vi "UI-Pore Diameter Detection.vi"(8 "error in (no error)":errorcluster caption="错误输入（无错误）", 11 "名称或相对路径":string="Template Program") -> (0 "error in (no error) 2":errorcluster caption="错误输入（无错误）")   [LabVIEW 2017]
uses:
  Picture/SaveButtom.ctl
  <vilib>/vision/Measure.llb/Edge Options.ctl
  <vilib>/vision/Measure.llb/Edge Polarity.ctl
  Global System.vi
  <vilib>/Utility/xml.llb/Read From XML File(string).vi
  <vilib>/Utility/xml.llb/Write to XML File(string).vi
panel:
  out "添加的路径 2":path
  out "计数器":dbl
  in  "启动200自动":bool
  out "孔径规格":T1
  out "原始图像 2":T2(plugin-control)
  in  "获取ROI":bool
  in  "GRR测试":bool
  in  "200测试":bool
  in  "采图按钮":bool
  in  "图像实时显示":bool
  out "添加的路径":path
  in  "刷新":bool
  in  "测试按钮":bool
  in  "保存按钮":bool
  in  "Main":enum32{"主参数", "计算圆心参数 ", "测试效果"}(tab)
  in  "ParamsUI":T3={"IsNorImage"=TRUE, "Exposure Values"=100289, "ImagePath"=path "C:/Users/hedongpo/Desktop/514-hdp/Alignment Assemble System/Test Picture/B/3.bmp"} caption="参数界面" {"Exposure Values" scale=0.0..200000.0}
  in  "ParamsUI 内圆":T7={"圆参数1"={"Search  Direction"=0, "Edge Options"={"Edge Polarity"=0, "Kernel Size"=3, "Width"=3, "Minimum Edge Strength"=50.0, "Interpolation Type"=enum."Bilinear Fixed", "Data Processing Method"=enum."Average"}, "Show Search Area"=TRUE, "Show Search Lines"=TRUE, "Show Edges Found"=TRUE, "Show Result"=TRUE, "Search Area Color"=65280, "Search Lines Color"=255, "Edge Locations Color"=16776960, "Result Color"=16711680, "Overlay Group Name"=""}, "圆参数"={"Process"=enum."Get First Edge", "Step Size"=1, "Max Pixel Radius"=3}, "圆环ROI设定"={"Center X"=1717, "Center Y"=1486, "Inner Radius"=327, "Outer Radius"=1645, "Start Angle"=0.0, "End Angle"=0.0}, "Show Search Area"=TRUE, "Show Search Lines"=TRUE, "Show Edges Found"=TRUE, "Show Result"=TRUE, "200次模板表格"=path "C:/Users/Administrator/Desktop/GRR模板/Test.xlsx", "GRR模板表格"=path "C:/Users/Administrator/Desktop/GRR模板/Test.xlsx", "孔径规格"={"孔径上限"="0.014", "孔径标准值"="1.1", "孔径下限"="0"}} caption="参数界面" {"圆环ROI设定"."End Angle" min=-90.0 max=90.0 step=1.0 format="%.2f"; "圆环ROI设定"."Start Angle" min=-90.0 max=90.0 step=1.0 format="%.2f"; "圆环ROI设定"."Center X" scale=0.0..1024.0; "圆参数1"."Search  Direction" items=["Outside to Inside", "Inside to Outside"]; "圆参数1"."Edge Options"."Edge Polarity" items=["All Edges", "Rising Edges", "Falling Edges"]; "圆参数1"."Edge Options"."Minimum Edge Strength" format="%.2f"; "圆参数1"."Edge Options"."Width" step=2; "圆参数1"."Edge Options"."Kernel Size" step=2}
  in  "测试历史记录":string[][](table)=[["", ""]]
  in  "测试结果":string[][](table)=[["", ""]]
  out "原始图像":T2(plugin-control)
  out "路径输出":path
  in  "Vision Paramter Save Buttom":T8
  out "system time":string
  in  "取消按钮":bool
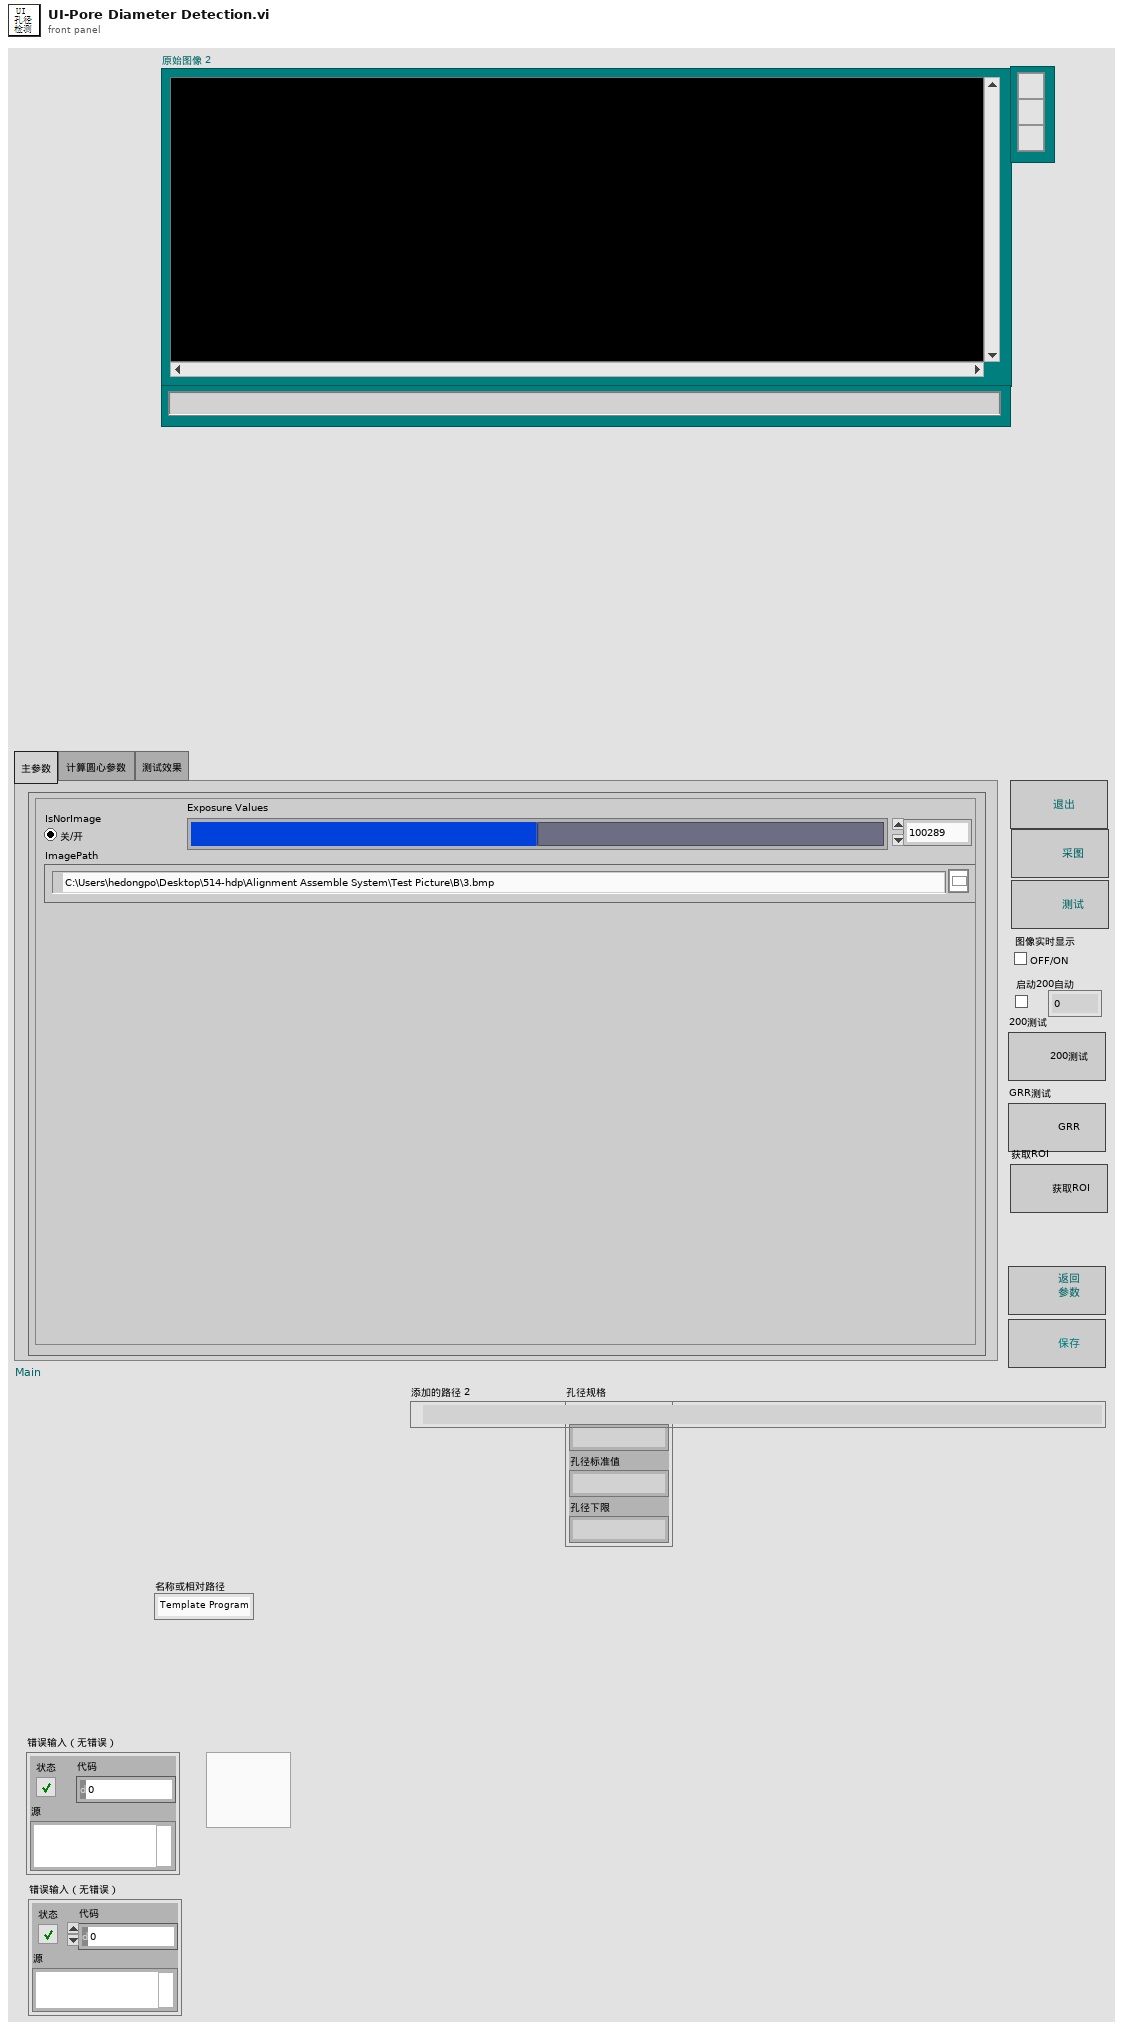
[diagram p1: front panel]
types:
  T1 = cluster{"孔径上限":string, "孔径标准值":string, "孔径下限":string}
  T2 = typedef "IMAQ Image.ctl" = refnum<image>
  T3 = cluster{"IsNorImage":bool, "Exposure Values":u32, "ImagePath":path}
  T4 = typedef "Edge Options.ctl" = cluster{"Edge Polarity":T5, "Kernel Size":u32, "Width":u32, "Minimum Edge Strength":sgl, "Interpolation Type":enum32{"Zero Order", "Bilinear", "Quadratic", "Cubic", "Bilinear Fixed"}, "Data Processing Method":enum32{"Average", "Median"}}
  T5 = typedef "Edge Polarity.ctl" = u32
  T6 = typedef "IMAQ Circle" = cluster{"Center X":i32, "Center Y":i32, "Inner Radius":i32, "Outer Radius":i32, "Start Angle":dbl, "End Angle":dbl}
  T7 = cluster{"圆参数1":cluster{"Search  Direction":u32, "Edge Options":T4, "Show Search Area":bool, "Show Search Lines":bool, "Show Edges Found":bool, "Show Result":bool, "Search Area Color":u32, "Search Lines Color":u32, "Edge Locations Color":u32, "Result Color":u32, "Overlay Group Name":string}, "圆参数":cluster{"Process":enum16{"Get First Edge", "Get First + Last Edge", "Get All Edges", "Get Best Edge"}, "Step Size":i32, "Max Pixel Radius":i32}, "圆环ROI设定":T6, "Show Search Area":bool, "Show Search Lines":bool, "Show Edges Found":bool, "Show Result":bool, "200次模板表格":path, "GRR模板表格":path, "孔径规格":cluster{"孔径上限":string, "孔径标准值":string, "孔径下限":string}}
  T8 = typedef "SaveButtom.ctl" = bool
  T9 = cluster{"index":i32, "this vi":refnum<vi>, "error out":errorcluster}
  T10 = cluster{"master data":string, "priority":u16, "secondary data":string[]}
  T11 = cluster{"case name":string[], "queue array":refnum<queue>[]}
  T12 = cluster{"Search  Direction":u32, "Edge Options":T4, "Show Search Area":bool, "Show Search Lines":bool, "Show Edges Found":bool, "Show Result":bool, "Search Area Color":u32, "Search Lines Color":u32, "Edge Locations Color":u32, "Result Color":u32, "Overlay Group Name":string}
  T13 = cluster{"Process":enum16{"Get First Edge", "Get First + Last Edge", "Get All Edges", "Get Best Edge"}, "Step Size":i32, "Max Pixel Radius":i32}
  T14 = typedef "ROI Descriptor" = cluster{"Global Rectangle":i32[], "Contours":cluster{"ID":enum32{"External", "Internal"}, "Type":u32, "Coordinates":i32[]}[]}
  T15 = cluster{"Center (Pixels)":cluster{"X":sgl, "Y":sgl}, "Radius (Pixels)":dbl, "Center (Real-World)":cluster{"X":sgl, "Y":sgl}, "Radius (Real-World)":dbl, "Roundness (Real-World)":dbl, "Average Strength":dbl, "Average SNR (dB)":dbl}
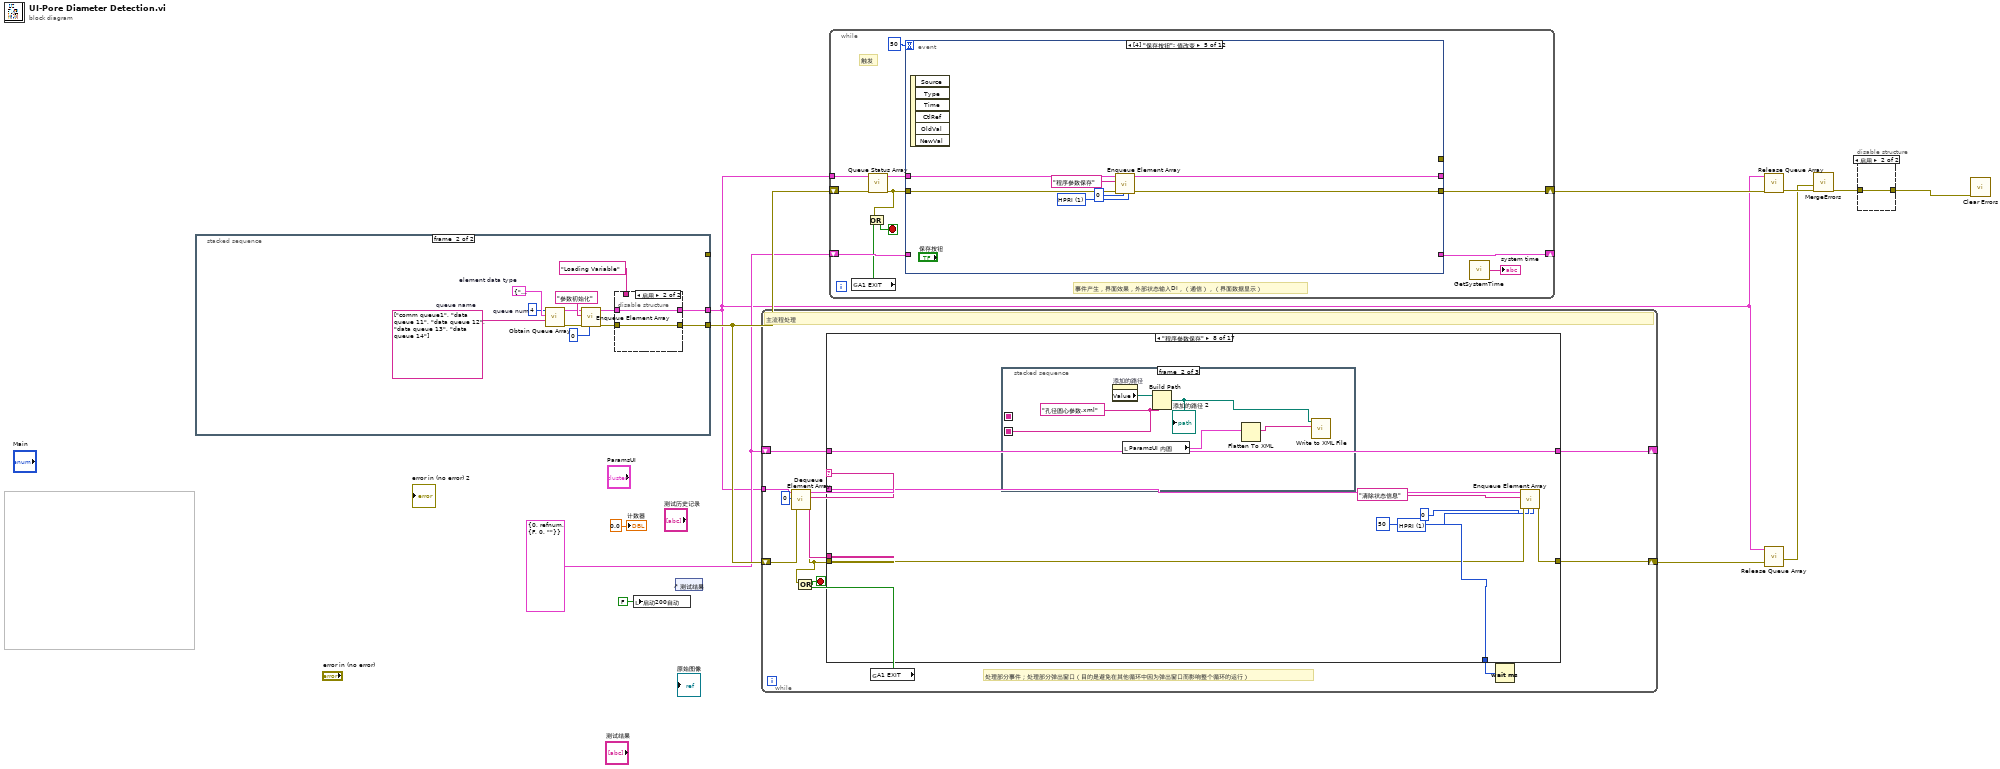
[diagram p0: block diagram]
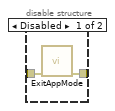
[diagram p2: hidden frame]
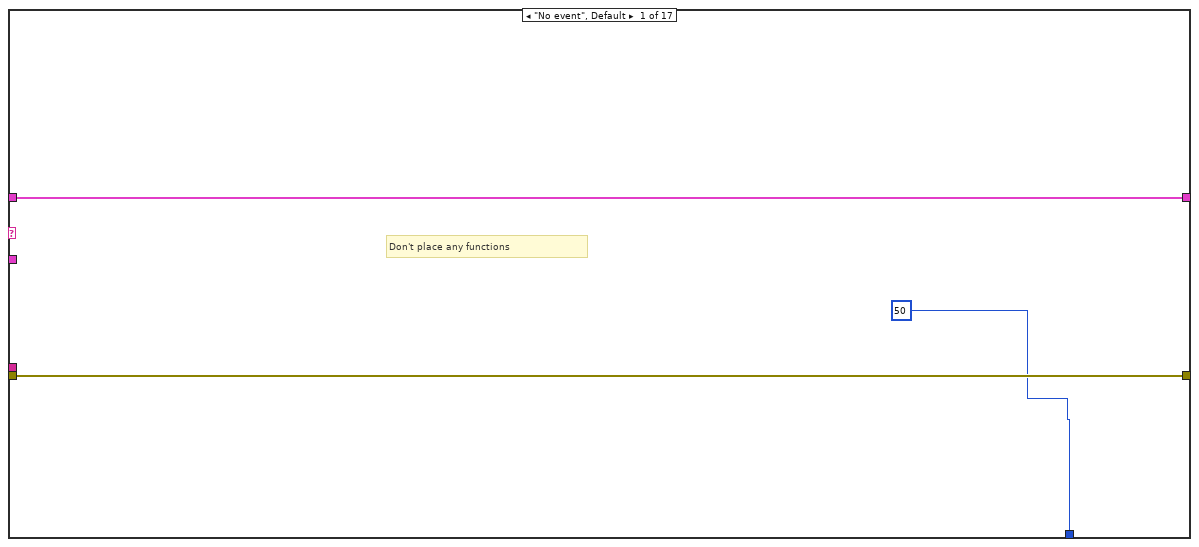
[diagram p3: hidden frame]
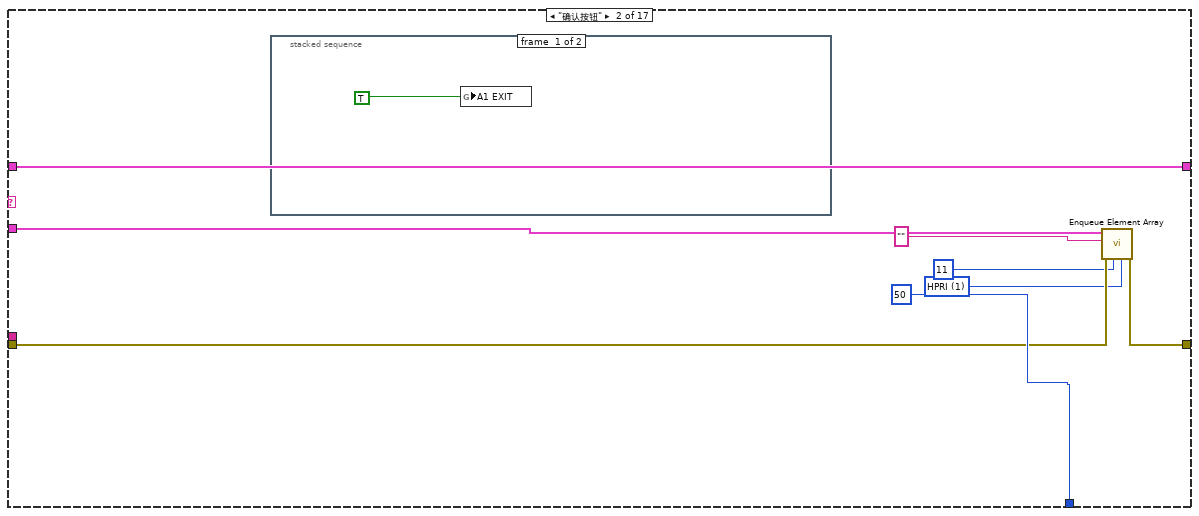
[diagram p4: hidden frame]
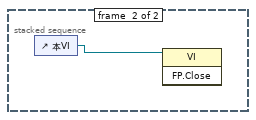
[diagram p5: hidden frame]
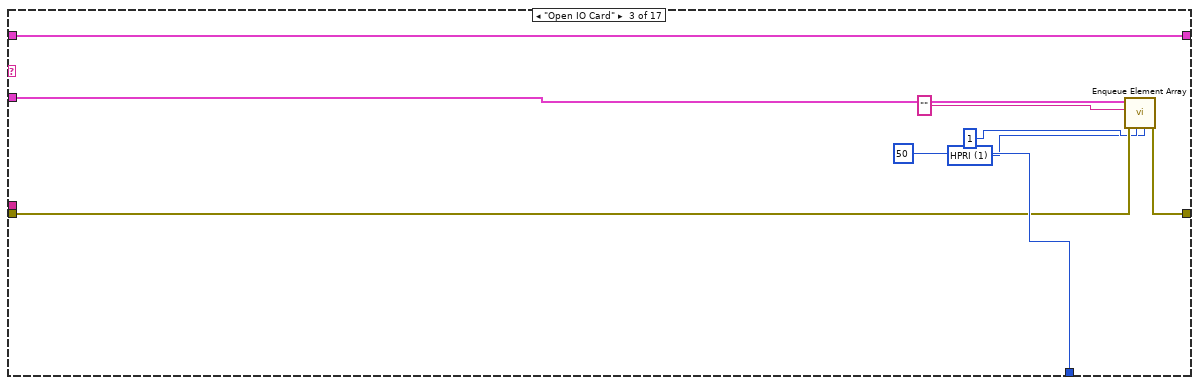
[diagram p6: hidden frame]
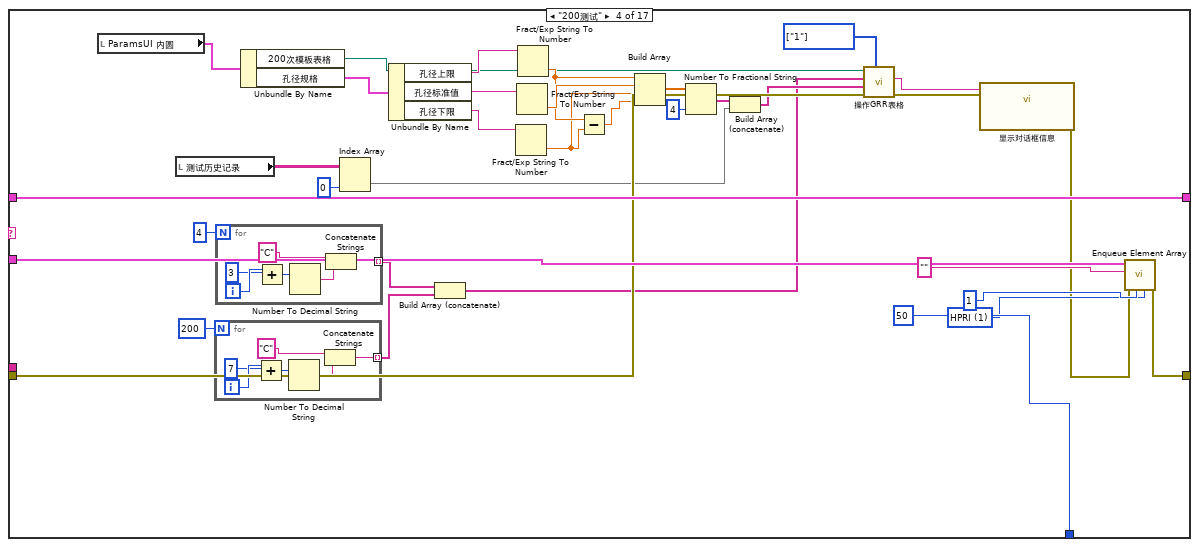
[diagram p7: hidden frame]
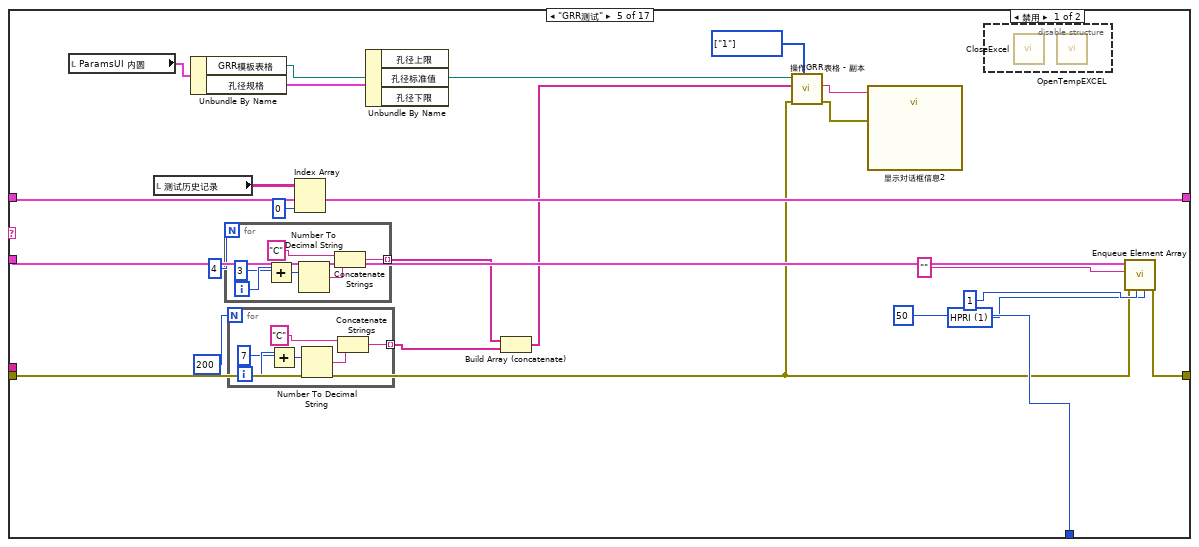
[diagram p8: hidden frame]
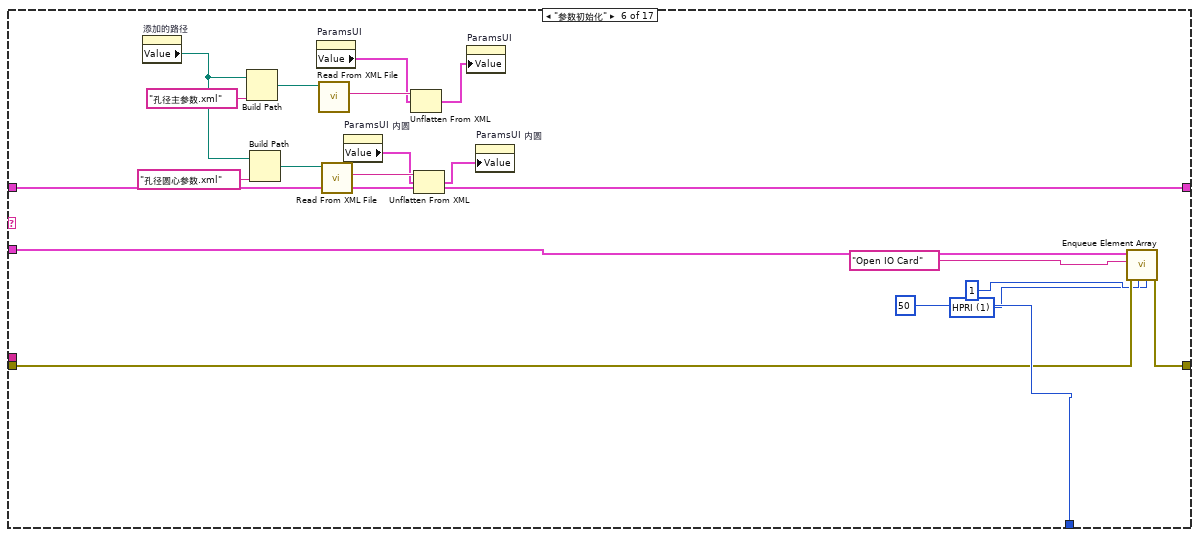
[diagram p10: hidden frame]
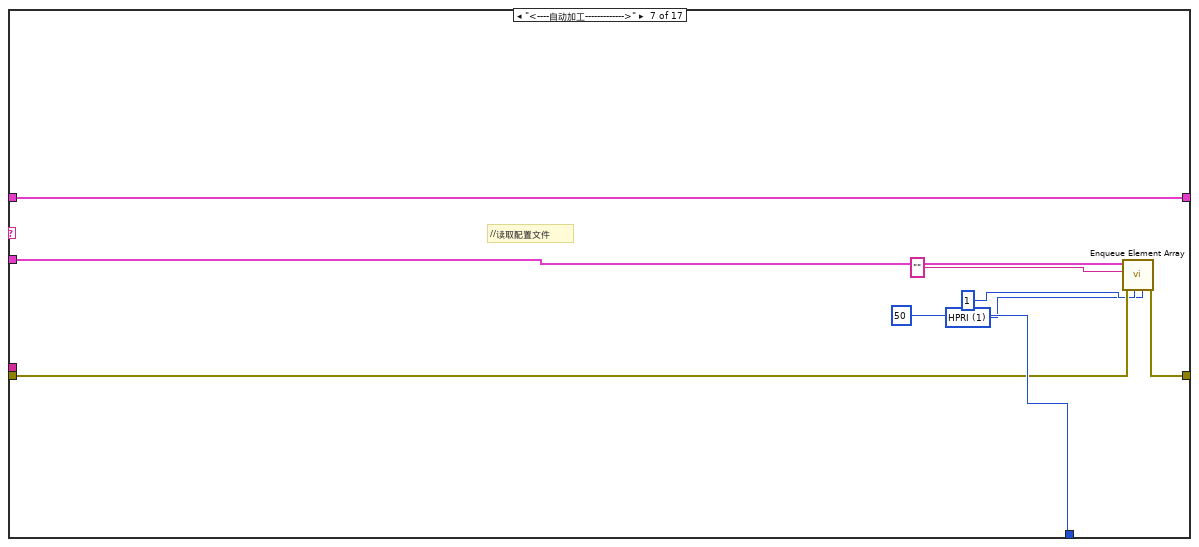
[diagram p11: hidden frame]
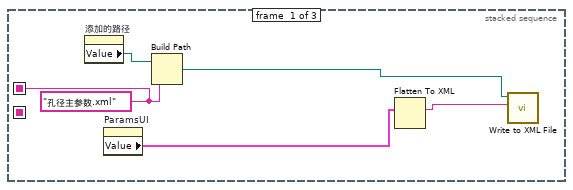
[diagram p12: hidden frame]
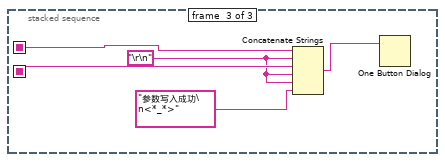
[diagram p13: hidden frame]
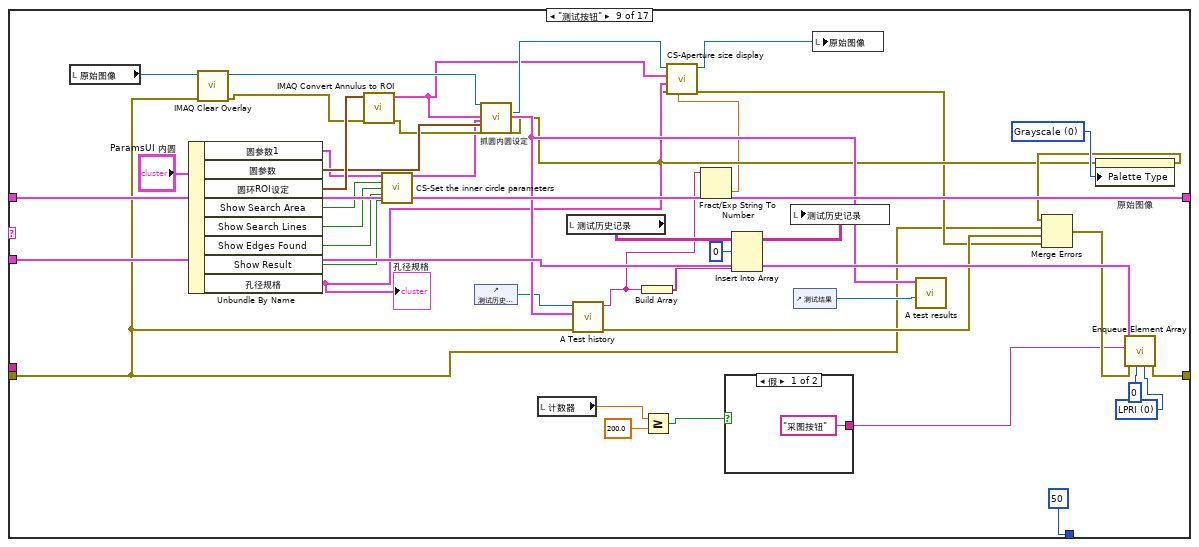
[diagram p14: hidden frame]
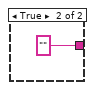
[diagram p15: hidden frame]
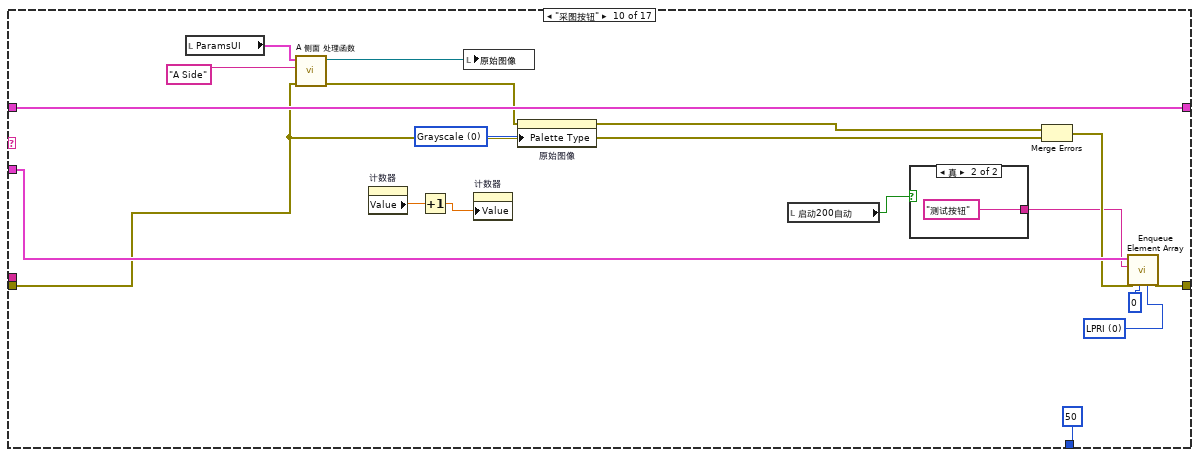
[diagram p16: hidden frame]
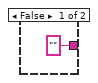
[diagram p17: hidden frame]
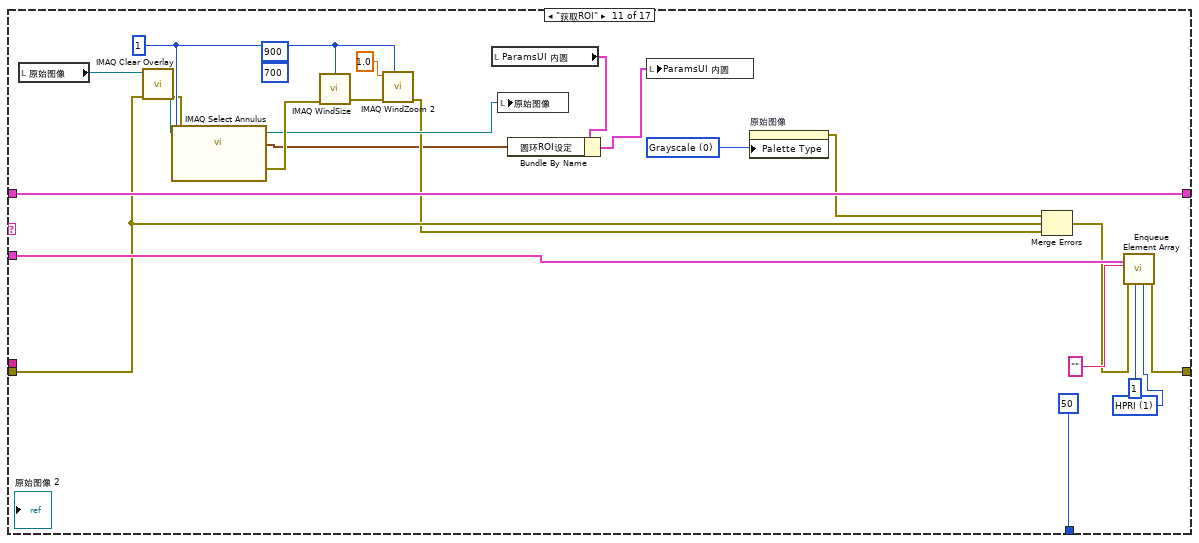
[diagram p18: hidden frame]
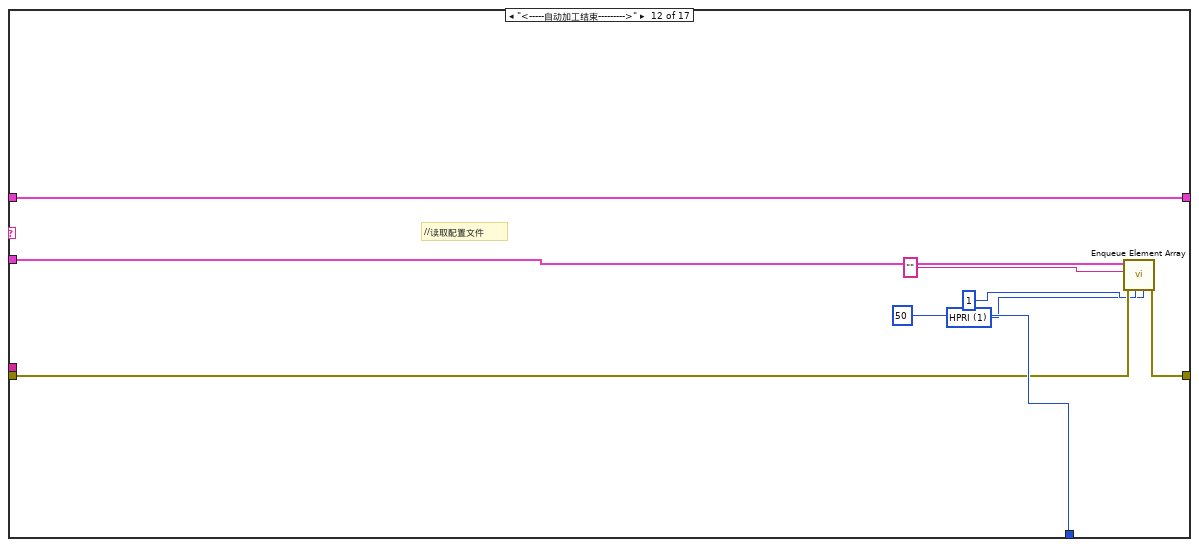
[diagram p19: hidden frame]
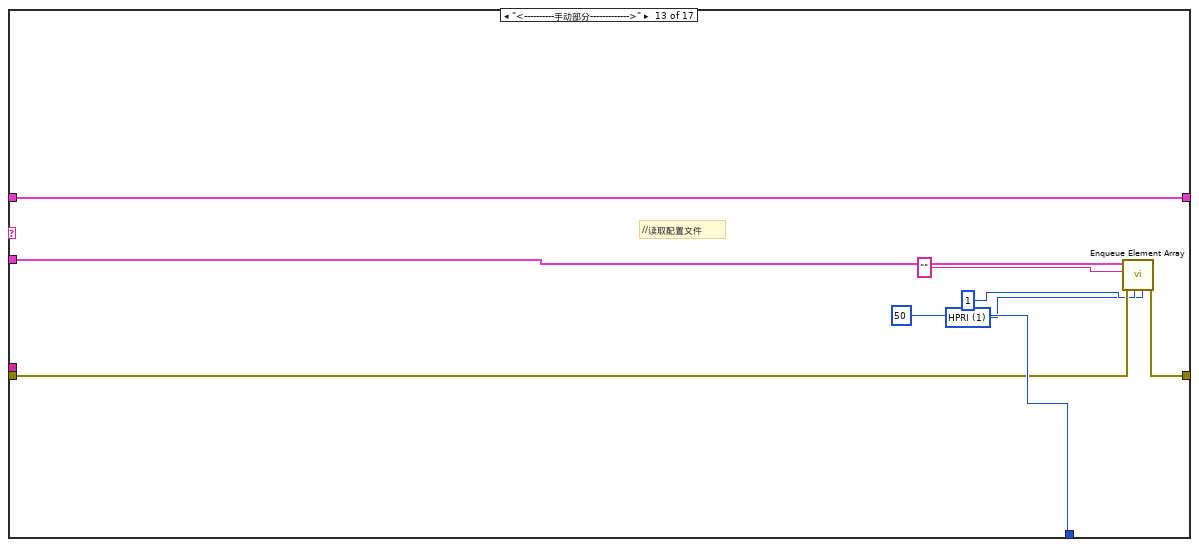
[diagram p20: hidden frame]
diagram:
  w6 = T9 {"index"=0, "this vi"=refnum, "error out"={"status"=FALSE, "code"=0, "source"=""}} ("parameter buffer")
  n1 = stacked-sequence {
    tunnel: [w19 _] -> _
    tunnel: [_ w23] -> w7
    tunnel: [_ w22] -> w3
    frame #0 {
      n2 = global read "Global System.vi" "ref path"() -> (w17:path)
      n3 = property on="Main" class="TabCtl (严格)"("Value"=enum32{"主参数", "计算圆心参数 ", "测试效果"}."主参数" ("Main")) -> ()  [unwired: 2 in, 2 out]
      n4 = Build Path(base path=w17, name or relative path="Template Program" ("名称或相对路径")) -> (appended path=w15:path)
      n5 = Build Path(base path=w15, name or relative path="名称或相对路径") -> (appended path=w21:path)
      "添加的路径" <- w21
      n6 = List Folder(path=w21) -> (path out=→"路径输出":path, error out=w19:errorcluster)  [unwired: 3 in, 2 out]
      n7 = local write "测试历史记录"(string[][] []) -> ()
      n8 = local write "图像实时显示"(FALSE ("图像实时显示")) -> ()
    }
    frame #1 {
      w31 = string[] ["comm queue1", "data queue 11", "data queue 12", "data queue 13", "data queue 14"]  # queue name
      w32 = 4  # queue num
      w33 = T10 {"master data"="", "priority"=0, "secondary data"=[]}  # element data type
      n9 = call "Obtain Queue Array.vi"("queue name"=w31, "element data type"=w33, "queue num"=w32) -> ("error out"=w27:errorcluster, "queue out"=w28:T11)  [unwired: 2 in, 1 out]
      n10 = call "Enqueue Element Array.vi"("queue index"=0, "error in"=w27, "master data"="参数初始化", "queue in"=w28) -> ("error out"=w26:errorcluster, "queue out"=w25:T11)  [unwired: 6 in]
      n11 = disable-structure shown="启用" {
        disable-tunnel: w26 -> [w39 w40]
        disable-tunnel: w25 -> [w38 w41]
        disable-tunnel: "Loading Variable" ("master data") -> [w37 _]
        disable-tunnel: [w35 w40] -> w23
        disable-tunnel: [w34 w41] -> w22
        frame Disabled {
          n12 = call "Enqueue Element Array.vi"("queue index"=12, "error in"=w39, "master data"=w37, "queue in"=w38) -> ("error out"=w35:errorcluster, "queue out"=w34:T11)  [unwired: 6 in]
        }
        frame Enabled {
        }
      }
    }
  }
  n13 = local write "启动200自动"(FALSE ("启动200自动")) -> ()
  n14 = control-ref of="测试结果"() -> ()  [unwired: 1 out]
  n15 = while {
    shift-right: [w54] -> w5
    shift-left: w7 -> [w45]
    shift-right: [w51] -> _
    shift-left: w6 -> [w52]
    tunnel: w3 -> [w47]
    stop <- w42 stop-if-true
    # "处理部分事件；处理部分弹出窗口（目的是避免在其他循环中因为弹出窗口而影响整个循环的运行）"
    # "主流程处理"
    n16 = call "Dequeue Element Array.vi"("queue in"=w47, "queue index"=0, "error in"=w45) -> ("queue out"=w50:T11, "master data"=w49:string, "secondary data"=w48:string[], "error out"=w44:errorcluster)  [unwired: 2 in, 1 out]
    n17 = case shown="\"程序参数保存\"" w49 {
      tunnel: w50 -> [_ w64 w74 w108 w141 w172 w180 w182 w246 w266 w291 w299 w307 w315 w323 w331 w337]
      tunnel: w44 -> [w56 w60 w70 w102 w122 w169 w176 w186 w214 w254 w274 w295 w303 w311 w319 w327 w334]
      tunnel: [w56 w63 w73 w107 w140 w171 w179 w188 w245 w265 w290 w298 w306 w314 w322 w330 w345] -> w54
      tunnel: [50 50 50 50 50 50 50 50 50 50 50 50 50 50 50 50 50] -> w53
      tunnel: w52 -> [w57 w61 w71 w105 w138 w166 w177 w183 w242 w262 w286 w296 w304 w312 w320 w328 w343]
      tunnel: [w57 w61 w71 w105 w138 w166 w177 w183 w242 w262 w286 w296 w304 w312 w320 w328 w343] -> w51
      tunnel: w48 -> [_ _ _ _ _ _ _ _ _ _ _ _ _ _ _ _ _]
      frame "No event", Default {
        # "Don't place any functions"
      }
      frame "确认按钮" {
        w58 = u16 1 items=["HPRI"=1, "LPRI"=0] ("priority")
        n18 = stacked-sequence {
          frame #0 {
            n19 = global write "Global System.vi" "A1 EXIT"(TRUE ("EXIT")) -> ()
          }
          frame #1 {
            n20 = control-ref of="本VI"() -> (w67:refnum<vi>)
            n21 = invoke class="VI" method="FP.Close"(reference=w67) -> ()  [unwired: 2 in, 3 out]
          }
        }
        n22 = call "Enqueue Element Array.vi"("priority"=w58, "queue index"=11, "error in"=w60, "master data"="" ("Element 1"), "queue in"=w64) -> ("error out"=w63:errorcluster)  [unwired: 5 in, 1 out]
      }
      frame "Open IO Card" {
        w68 = u16 1 items=["HPRI"=1, "LPRI"=0] ("priority")
        n23 = call "Enqueue Element Array.vi"("priority"=w68, "queue index"=1, "error in"=w70, "master data"="" ("Element 1"), "queue in"=w74) -> ("error out"=w73:errorcluster)  [unwired: 5 in, 1 out]
      }
      frame "200测试" {
        w76 = enum16{"0", "1", "2"}[] [enum."1"] items=["0", "1", "2"] ("表单")
        w103 = u16 1 items=["HPRI"=1, "LPRI"=0] ("priority")
        n24 = local read "ParamsUI 内圆"() -> (w98:T7)
        n25 = local read "测试历史记录"() -> (w100:string[][])
        n26 = for {
          N: 200 -> [_]
          tunnel: [w110] -> w81 mode=indexing
          i -> [w114]
          n27 = Add(x=w114, y=7) -> (x+y=w112:i32)
          n28 = Number To Decimal String(number=w112) -> (decimal integer string=w111:string)  [unwired: 1 in]
          n29 = Concatenate Strings("C", w111) -> (w110:string)
        }
        n30 = for {
          N: 4 -> [_]
          tunnel: [w116] -> w82 mode=indexing
          i -> [w120]
          n31 = Add(x=w120, y=3) -> (x+y=w118:i32)
          n32 = Number To Decimal String(number=w118) -> (decimal integer string=w117:string)  [unwired: 1 in]
          n33 = Concatenate Strings("C", w117) -> (w116:string)
        }
        n34 = Unbundle By Name(w98) -> ("200次模板表格"=w79:path, "孔径规格"=w97:T1)
        n35 = Index Array(array=w100, index (col)=0 ("禁用的索引 (列)")) -> (element=w86:string[])  [unwired: 1 in]
        n36 = Unbundle By Name(w97) -> ("孔径上限"=w96:string, "孔径标准值"=w95:string, "孔径下限"=w94:string)
        n37 = Build Array (concatenate)(w82, w81) -> (w80:string[])
        n38 = Fract/Exp String To Number(string=w94) -> (number=w91:dbl)  [unwired: 3 in, 1 out]
        n39 = Fract/Exp String To Number(string=w95) -> (number=w93:dbl)  [unwired: 3 in, 1 out]
        n40 = Fract/Exp String To Number(string=w96) -> (number=w92:dbl)  [unwired: 3 in, 1 out]
        n41 = Subtract(x=w92, y=w91) -> (x-y=w90:dbl)
        n42 = Build Array(w92, w93, w91, w90) -> (w89:dbl[])
        n43 = Number To Fractional String(number=w89, precision (6)=i16 4 ("精度(6)")) -> (F-format string=w87:string[])  [unwired: 2 in]
        n44 = Build Array (concatenate)(w87, w86) -> (w85:string[])
        n45 = call "操作GRR表格.vi"("表单"=w76, "错误输入（无错误）"=w102, "数据"=w85, "位置"=w80, "路径"=w79) -> ("错误输出"=w101:errorcluster, "number"=w77:string)  [unwired: 4 in, 1 out]
        n46 = call "显示对话框信息"("error in (no error)"=w101, "Message"=w77) -> ("error out"=w78:errorcluster)  [unwired: 8 in, 1 out]
        n47 = call "Enqueue Element Array.vi"("priority"=w103, "queue index"=1, "error in"=w78, "master data"="" ("Element 1"), "queue in"=w108) -> ("error out"=w107:errorcluster)  [unwired: 5 in, 1 out]
      }
      frame "GRR测试" {
        w130 = enum16{"0", "1", "2"}[] [enum."1"] items=["0", "1", "2"] ("表单")
        w136 = u16 1 items=["HPRI"=1, "LPRI"=0] ("priority")
        n48 = local read "ParamsUI 内圆"() -> (w133:T7)
        n49 = local read "测试历史记录"() -> (w126:string[][])
        n50 = Unbundle By Name(w133) -> ("GRR模板表格"=w131:path, "孔径规格"=w132:T1)
        n51 = for {
          N: 4 -> [_]
          tunnel: [w149] -> w129 mode=indexing
          i -> [w153]
          n52 = Add(x=w153, y=3) -> (x+y=w151:i32)
          n53 = Number To Decimal String(number=w151) -> (decimal integer string=w150:string)  [unwired: 1 in]
          n54 = Concatenate Strings("C", w150) -> (w149:string)
        }
        n55 = for {
          N: 200 -> [_]
          tunnel: [w143] -> w128 mode=indexing
          i -> [w147]
          n56 = Add(x=w147, y=7) -> (x+y=w145:i32)
          n57 = Number To Decimal String(number=w145) -> (decimal integer string=w144:string)  [unwired: 1 in]
          n58 = Concatenate Strings("C", w144) -> (w143:string)
        }
        n59 = Index Array(array=w126, index (col)=0 ("禁用的索引 (列)")) -> ()  [unwired: 1 in, 1 out]
        n60 = Unbundle By Name(w132) -> ()  [unwired: 3 out]
        n61 = Build Array (concatenate)(w129, w128) -> (w127:string[])
        n62 = call "操作GRR表格 - 副本.vi"("表单"=w130, "错误输入（无错误）"=w122, "位置"=w127, "路径"=w131) -> ("错误输出"=w123:errorcluster, "number"=w124:string)  [unwired: 5 in, 1 out]
        n63 = call "显示对话框信息2"("error in (no error)"=w123, "Message"=w124) -> ()  [unwired: 8 in, 2 out]
        n64 = disable-structure shown="禁用" {
          frame Disabled {
            n65 = call "CloseExcel.vi"() -> ()  [unwired: 11 in, 1 out]
            n66 = call "OpenTempEXCEL.vi"() -> ()  [unwired: 10 in, 2 out]
          }
          frame Enabled {
          }
        }
        n67 = call "Enqueue Element Array.vi"("priority"=w136, "queue index"=1, "error in"=w122, "master data"="" ("Element 1"), "queue in"=w141) -> ("error out"=w140:errorcluster)  [unwired: 5 in, 1 out]
      }
      frame "参数初始化" {
        w167 = u16 1 items=["HPRI"=1, "LPRI"=0] ("priority")
        n68 = property on="添加的路径" class="Path"() -> ("Value"=w160:path)  [unwired: 2 in, 2 out]
        n69 = Build Path(base path=w160, name or relative path="孔径主参数.xml" ("名称或相对路径")) -> (appended path=w164:path)
        n70 = Build Path(base path=w160, name or relative path="孔径圆心参数.xml" ("名称或相对路径")) -> (appended path=w158:path)
        n71 = property on="ParamsUI" class="Clust (严格)"() -> ("Value"=w162:T3)  [unwired: 2 in, 2 out]
        n72 = call-poly <vilib>:"Read From XML File.vi"("XML File Path"=w164) -> ("XML Elements"=w163:string)  [unwired: 8 in, 2 out]
        n73 = call-poly <vilib>:"Read From XML File.vi"("XML File Path"=w158) -> ("XML Elements"=w159:string)  [unwired: 8 in, 2 out]
        n74 = property on="ParamsUI 内圆" class="Clust (严格)"() -> ("Value"=w156:T7)  [unwired: 2 in, 2 out]
        n75 = Unflatten From XML(xml string=w163, type=w162) -> (value=w161:T3)  [unwired: 1 in, 1 out]
        n76 = Unflatten From XML(xml string=w159, type=w156) -> (value=w155:T7)  [unwired: 1 in, 1 out]
        n77 = property on="ParamsUI" class="Clust (严格)"("Value"=w161) -> ()  [unwired: 2 in, 2 out]
        n78 = property on="ParamsUI 内圆" class="Clust (严格)"("Value"=w155) -> ()  [unwired: 2 in, 2 out]
        n79 = call "Enqueue Element Array.vi"("priority"=w167, "queue index"=1, "error in"=w169, "master data"="Open IO Card" ("Element 1"), "queue in"=w172) -> ("error out"=w171:errorcluster)  [unwired: 5 in, 1 out]
      }
      frame "<----自动加工------------->" {
        w174 = u16 1 items=["HPRI"=1, "LPRI"=0] ("priority")
        # "//读取配置文件"
        n80 = call "Enqueue Element Array.vi"("priority"=w174, "queue index"=1, "error in"=w176, "master data"="" ("Element 1"), "queue in"=w180) -> ("error out"=w179:errorcluster)  [unwired: 5 in, 1 out]
      }
      frame "程序参数保存" {
        w184 = u16 1 items=["HPRI"=1, "LPRI"=0] ("priority")
        n81 = stacked-sequence {
          seq-local: [w190 _ _] -> [_ _ w203]
          seq-local: [_ w195 _] -> [_ _ w201]
          frame #0 {
            w190 = "孔径主参数.xml" ("名称或相对路径")
            n82 = property on="添加的路径" class="Path"() -> ("Value"=w194:path)  [unwired: 2 in, 2 out]
            n83 = property on="ParamsUI" class="Clust (严格)"() -> ("Value"=w193:T3)  [unwired: 2 in, 2 out]
            n84 = Build Path(base path=w194, name or relative path=w190) -> (appended path=w191:path)
            n85 = Flatten To XML(anything=w193) -> (xml string=w192:string)
            n86 = call-poly <vilib>:"Write to XML File.vi"("XML Input"=w192, "XML File Path"=w191) -> ()  [unwired: 7 in, 3 out]
          }
          frame #1 {
            w195 = "孔径圆心参数.xml" ("名称或相对路径")
            n87 = property on="添加的路径" class="Path"() -> ("Value"=w199:path)  [unwired: 2 in, 2 out]
            n88 = local read "ParamsUI 内圆"() -> (w196:T7)
            n89 = Build Path(base path=w199, name or relative path=w195) -> (appended path=w197:path)
            "添加的路径 2" <- w197
            n90 = Flatten To XML(anything=w196) -> (xml string=w198:string)
            n91 = call-poly <vilib>:"Write to XML File.vi"("XML Input"=w198, "XML File Path"=w197) -> ()  [unwired: 7 in, 3 out]
          }
          frame #2 {
            w200 = "\r\n"
            n92 = Concatenate Strings(w203, w200, w201, w200, w200, "参数写入成功\n<*_*>" ("消息")) -> (w202:string)
            n93 = One Button Dialog(message=w202) -> ()  [unwired: 1 in, 1 out]
          }
        }
        n94 = call "Enqueue Element Array.vi"("priority"=w184, "queue index"=0, "error in"=w186, "master data"="清除状态信息" ("Element 1"), "queue in"=w182) -> ("error out"=w188:errorcluster)  [unwired: 5 in, 1 out]
      }
      frame "测试按钮" {
        w241 = u32 0 items=["Grayscale", "Binary", "Gradient", "Rainbow", "Temperature", "User Defined", "Binary 16 Bit", "Gradient 16 Bit", "Rainbow 16 Bit", "Temperature 16 Bit", "User Defined 16 Bit"] ("Palette:Palette Type")
        w243 = u16 0 items=["HPRI"=1, "LPRI"=0] ("priority")
        n95 = local read "原始图像"() -> (w223:T2)
        n96 = Unbundle By Name("ParamsUI 内圆") -> ("圆参数1"=w212:T12, "圆参数"=w236:T13, "圆环ROI设定"=w237:T6, "Show Search Area"=w235:bool, "Show Search Lines"=w234:bool, "Show Edges Found"=w233:bool, "Show Result"=w232:bool, "孔径规格"=w221:T1)
        "孔径规格" <- w221
        n97 = call "IMAQ Clear Overlay"("error in (no error)"=w214, "Image"=w223) -> ("error out"=w213:errorcluster, "Image Out"=w215:T2)  [unwired: 8 in]
        n98 = call "IMAQ Convert Annulus to ROI"("error in (no error)"=w213, "Annulus"=w237) -> ("error out"=w222:errorcluster, "ROI Descriptor"=w211:T14)  [unwired: 7 in]
        n99 = call "CS-Set the inner circle parameters.vi"("内圆参数in"=w212, "Show Search Area"=w235, "Show Search Lines"=w234, "Show Edges Found"=w233, "Show Result"=w232) -> ("our"=w210:T12)  [unwired: 10 in]
        n100 = control-ref of="测试历史记录"() -> (w224:refnum<vi>)
        n101 = call "抓圆内圆设定"("Image In"=w215, "ROI Descriptor (Find Circular Edge 1)"=w211, "Options (Find Circular Edge 1)"=w210, "Circle Fit Options (Find Circular Edge 1)"=w236, "error in"=w222) -> ("Image Out"=w218:T2, "Fitted Circle (Find Circular Edge 1)"=w229:T15, "error out"=w220:errorcluster)  [unwired: 20 in]
        n102 = local read "计数器"() -> (w209:dbl)
        n103 = local read "测试历史记录"() -> (w231:string[][])
        n104 = call "A Test history.vi"("错误输入（无错误）"=w214, "Fitted Circle (Find Circular Edge 1)"=w229, "Tbl引用句柄"=w224) -> ("错误输出"=w227:errorcluster, "F-格式字符串"=w216:string)  [unwired: 7 in]
        n105 = Build Array(w216) -> (w226:string[])
        n106 = Greater Or Equal?(x=w209, y=200.0) -> (x >= y?=w207:bool)
        n107 = Fract/Exp String To Number(string=w216) -> (number=w205:dbl)  [unwired: 3 in, 1 out]
        n108 = call "CS-Aperture size display.vi"("实际孔径"=w205, "error in (no error)"=w220, "孔径规格"=w221, "ROI Descriptor"=w211, "原始图像 IN"=w218) -> ("error out"=w219:errorcluster, "原始图像 OUT"=w217:T2)  [unwired: 2 in, 3 out]
        n109 = case shown="假" w207 {
          tunnel: ["采图按钮" ("Element 1") "" ("Element 1")] -> w206
          frame False {
          }
          frame True {
          }
        }
        n110 = Insert Into Array(array=w231, index (row)=0 ("索引 (行)"), new element=w226) -> (w228:string[][])  [unwired: 1 in]
        n111 = local write "测试历史记录"(w228) -> ()
        n112 = control-ref of="测试结果"() -> (w225:refnum<vi>)
        n113 = local write "原始图像"(w217) -> ()
        n114 = call "A test results.vi"("Fitted Circle (Find Circular Edge 1)"=w229, "Tbl引用句柄"=w225) -> ()  [unwired: 8 in, 1 out]
        n115 = property on="原始图像" class="ImageControl"(error in=w220, "Palette Type"=w241) -> (error out=w240:errorcluster)  [unwired: 1 in, 1 out]
        n116 = Merge Errors(w240, w214, w227, w219) -> (w239:errorcluster)
        n117 = call "Enqueue Element Array.vi"("priority"=w243, "queue index"=0, "error in"=w239, "master data"=w206, "queue in"=w246) -> ("error out"=w245:errorcluster)  [unwired: 5 in, 1 out]
      }
      frame "采图按钮" {
        w260 = u32 0 items=["Grayscale", "Binary", "Gradient", "Rainbow", "Temperature", "User Defined", "Binary 16 Bit", "Gradient 16 Bit", "Rainbow 16 Bit", "Temperature 16 Bit", "User Defined 16 Bit"] ("Palette:Palette Type")
        w263 = u16 0 items=["HPRI"=1, "LPRI"=0] ("priority")
        n118 = local read "ParamsUI"() -> (w259:T3)
        n119 = call "A 侧面 处理函数.vi"("error in (no error)"=w254, "Image Name"="A Side", "ParamsUI"=w259) -> ("error out"=w255:errorcluster, "Image out"=w256:T2)  [unwired: 5 in, 2 out]
        n120 = property on="计数器" class="DigNum (严格)"() -> ("Value"=w251:dbl)  [unwired: 2 in, 2 out]
        n121 = Increment(x=w251) -> (x+1=w250:dbl)
        n122 = local write "原始图像"(w256) -> ()
        n123 = property on="计数器" class="DigNum (严格)"("Value"=w250) -> ()  [unwired: 2 in, 2 out]
        n124 = property on="原始图像" class="ImageControl"(error in=w255, "Palette Type"=w260) -> (error out=w258:errorcluster)  [unwired: 1 in, 1 out]
        n125 = local read "启动200自动"() -> (w253:bool)
        n126 = case shown="真" w253 {
          tunnel: ["" ("Element 1") "测试按钮" ("Element 1")] -> w252
          frame False {
          }
          frame True {
          }
        }
        n127 = Merge Errors(w258, w254) -> (w257:errorcluster)
        n128 = call "Enqueue Element Array.vi"("priority"=w263, "queue index"=0, "error in"=w257, "master data"=w252, "queue in"=w266) -> ("error out"=w265:errorcluster)  [unwired: 5 in, 1 out]
      }
      frame "获取ROI" {
        (unwired) 900 ("Width")
        (unwired) 700 ("Height")
        w281 = 1 ("Window Number (0...15)")
        w285 = u32 0 items=["Grayscale", "Binary", "Gradient", "Rainbow", "Temperature", "User Defined", "Binary 16 Bit", "Gradient 16 Bit", "Rainbow 16 Bit", "Temperature 16 Bit", "User Defined 16 Bit"] ("Palette:Palette Type")
        w287 = u16 1 items=["HPRI"=1, "LPRI"=0] ("priority")
        n129 = local read "原始图像"() -> (w276:T2)
        n130 = call "IMAQ Clear Overlay"("error in (no error)"=w274, "Image"=w276) -> ("error out"=w278:errorcluster, "Image Out"=w277:T2)  [unwired: 8 in]
        n131 = call "IMAQ Select Annulus"("Window Number (0...15)"=w281, "error in (no error)"=w278, "Image In"=w277) -> ("error out"=w282:errorcluster, "Annulus"=w270:T6, "Image Out (duplicate)"=w275:T2)  [unwired: 5 in, 1 out]
        n132 = call "IMAQ WindSize"("error in (no error)"=w282, "Window Number"=w281) -> ("error out"=w280:errorcluster)  [unwired: 4 in, 2 out]
        n133 = call "IMAQ WindZoom 2"("Window Number (0...15)"=w281, "error in (no error)"=w280, "Zoom Factor"=sgl 1.0) -> ("error out"=w273:errorcluster)  [unwired: 5 in, 3 out]
        n134 = local read "ParamsUI 内圆"() -> (w272:T7)
        n135 = local write "原始图像"(w275) -> ()
        n136 = Bundle By Name(cluster=w272, "圆环ROI设定"=w270) -> (w271:T7)
        n137 = local write "ParamsUI 内圆"(w271) -> ()
        n138 = property on="原始图像" class="ImageControl"("Palette Type"=w285) -> (error out=w284:errorcluster)  [unwired: 2 in, 1 out]
        n139 = Merge Errors(w284, w274, w273) -> (w283:errorcluster)
        n140 = call "Enqueue Element Array.vi"("priority"=w287, "queue index"=1, "error in"=w283, "master data"="" ("Element 1"), "queue in"=w291) -> ("error out"=w290:errorcluster)  [unwired: 5 in, 1 out]
      }
      frame "<-----自动加工结束--------->" {
        w293 = u16 1 items=["HPRI"=1, "LPRI"=0] ("priority")
        # "//读取配置文件"
        n141 = call "Enqueue Element Array.vi"("priority"=w293, "queue index"=1, "error in"=w295, "master data"="" ("Element 1"), "queue in"=w299) -> ("error out"=w298:errorcluster)  [unwired: 5 in, 1 out]
      }
      frame "<----------手动部分------------->" {
        w301 = u16 1 items=["HPRI"=1, "LPRI"=0] ("priority")
        # "//读取配置文件"
        n142 = call "Enqueue Element Array.vi"("priority"=w301, "queue index"=1, "error in"=w303, "master data"="" ("Element 1"), "queue in"=w307) -> ("error out"=w306:errorcluster)  [unwired: 5 in, 1 out]
      }
      frame "参数设置保存" {
        w309 = u16 1 items=["HPRI"=1, "LPRI"=0] ("priority")
        n143 = call "Enqueue Element Array.vi"("priority"=w309, "queue index"=1, "error in"=w311, "master data"="" ("Element 1"), "queue in"=w315) -> ("error out"=w314:errorcluster)  [unwired: 5 in, 1 out]
      }
      frame "200自动" {
        w317 = u16 0 items=["HPRI"=1, "LPRI"=0] ("priority")
        n144 = call "Enqueue Element Array.vi"("priority"=w317, "queue index"=0, "error in"=w319, "master data"="采图按钮" ("Element 1"), "queue in"=w323) -> ("error out"=w322:errorcluster)  [unwired: 5 in, 1 out]
      }
      frame "<--------------手动结束---------------->" {
        w325 = u16 1 items=["HPRI"=1, "LPRI"=0] ("priority")
        # "//读取配置文件"
        n145 = call "Enqueue Element Array.vi"("priority"=w325, "queue index"=1, "error in"=w327, "master data"="" ("Element 1"), "queue in"=w331) -> ("error out"=w330:errorcluster)  [unwired: 5 in, 1 out]
      }
      frame "*Emergency alarm" {
        w340 = u16 1 items=["HPRI"=1, "LPRI"=0] ("priority")
        w341 = u16 1 items=["HPRI"=1, "LPRI"=0] ("priority")
        # "发出处理急停信号的命令"
        # "发出处理急停信号的命令"
        n146 = call "Enqueue Element Array.vi"("priority"=w340, "queue index"=0, "error in"=w334, "master data"="" ("Element 1"), "queue in"=w337) -> ("error out"=w335:errorcluster, "queue out"=w336:T11)  [unwired: 5 in]
        n147 = call "SetTestInfoIndex.vi"("test info index"=13) -> ()
        n148 = call "Enqueue Element Array.vi"("priority"=w341, "queue index"=1, "error in"=w335, "master data"="" ("Element 1"), "queue in"=w336) -> ("error out"=w345:errorcluster)  [unwired: 5 in, 1 out]
      }
    }
    n149 = global read "Global System.vi" "A1 EXIT"() -> (w43:bool)
    n150 = Or(x=w44, y=w43) -> (x .or. y?=w42:bool)
    n151 = Wait (ms)(milliseconds to wait=w53) -> ()  [unwired: 1 out]
  }
  n152 = while {
    shift-right: [w350] -> w8
    shift-left: w7 -> [w354]
    shift-right: [w352] -> _
    shift-left: w6 -> [w353]
    tunnel: w3 -> [w356]
    stop <- w347 stop-if-true
    # "触发"
    # "事件产生，界面效果，外部状态输入DI，（通信），（界面数据显示）"
    n153 = global read "Global System.vi" "A1 EXIT"() -> (w348:bool)
    n154 = call "Queue Status Array.vi"("error in (no error)"=w354, "queue in"=w356) -> ("error out"=w349:errorcluster, "queue out"=w351:T11)  [unwired: 4 in]
    n155 = Or(x=w349, y=w348) -> (x .or. y?=w347:bool)
    n156 = event shown="[4] \"保存按钮\": 值改变" {
      selector: _ -> [_ _ _ _ _ _ _ _ _ _ _ _]
      dyn-events: _ -> [_ _ _ _ _ _ _ _ _ _ _ _]
      timeout: 50 -> [_ _ _ _ _ _ _ _ _ _ _ _]
      tunnel: w353 -> [w362 w376 _ _ _ _ _ _ _ _ _ _]
      tunnel: [w362 w376 _ _ _ _ _ _ _ _ _ _] -> w352
      tunnel: [errorcluster {"status"=FALSE, "code"=0, "source"=""} ("error out") _ _ _ _ _ _ _ _ _ _ _] -> _
      tunnel: w351 -> [w360 w375 w381 w388 w395 w404 w413 w423 w431 w439 w447 w455]
      tunnel: w349 -> [w358 w374 w380 w387 w394 w403 w412 w422 w430 w438 w446 w454]
      tunnel: [w358 w373 w378 w385 w392 w401 w410 w420 w428 w436 w444 w452] -> w350
      tunnel: [w360 w372 w379 w386 w393 w402 w411 w421 w429 w437 w445 w453] -> _
      event Timeout {
        # "不要在事件结构里面放入\"弹出窗口\"这样的VI保证该循环畅通无阻。"
        n157 = event-data() -> ()  [unwired: 1 in, 1 out]
        n158 = case shown="真" "图像实时显示" {
          tunnel: w358 -> [_ w365]
          frame False {
          }
          frame True {
            w366 = u32 0 items=["Grayscale", "Binary", "Gradient", "Rainbow", "Temperature", "User Defined", "Binary 16 Bit", "Gradient 16 Bit", "Rainbow 16 Bit", "Temperature 16 Bit", "User Defined 16 Bit"] ("Palette:Palette Type")
            n159 = local read "ParamsUI"() -> (w368:T3)
            n160 = call "Get aperture images.vi"("error in (no error)"=w365, "Image Name"="Curent", "ParamsUI"=w368) -> ("error out"=w364:errorcluster, "Image out"=w363:T2)  [unwired: 5 in, 2 out]
            n161 = local write "原始图像"(w363) -> ()
            n162 = property on="原始图像" class="ImageControl"(error in=w364, "Palette Type"=w366) -> ()  [unwired: 1 in, 2 out]
          }
        }
      }
      event Panel Close? {
        w370 = u16 1 items=["HPRI"=1, "LPRI"=0] ("priority")
        n163 = event-data() -> ()  [unwired: 1 in, 4 out]
        n164 = call "Enqueue Element Array.vi"("priority"=w370, "queue index"=0, "error in"=w374, "master data"="*Exit application", "queue in"=w375) -> ("error out"=w373:errorcluster, "queue out"=w372:T11)  [unwired: 5 in]
        n165 = event-data("Discard?"=TRUE) -> ()  [unwired: 1 in, 1 out]
      }
      event Value Change {
        w383 = u16 1 items=["HPRI"=1, "LPRI"=0] ("priority")
        n166 = event-data() -> ()  [unwired: 1 in, 6 out]
        n167 = call "Enqueue Element Array.vi"("priority"=w383, "queue index"=0, "error in"=w380, "master data"="Vision Paramter Save", "queue in"=w381) -> ("error out"=w378:errorcluster, "queue out"=w379:T11)  [unwired: 5 in]
      }
      event "取消按钮": Value Change {
        w390 = u16 1 items=["HPRI"=1, "LPRI"=0] ("priority")
        n168 = event-data() -> ()  [unwired: 1 in, 6 out]
        n169 = call "Enqueue Element Array.vi"("priority"=w390, "queue index"=0, "error in"=w387, "master data"="确认按钮", "queue in"=w388) -> ("error out"=w385:errorcluster, "queue out"=w386:T11)  [unwired: 5 in]
      }
      event "保存按钮": Value Change {
        w397 = u16 1 items=["HPRI"=1, "LPRI"=0] ("priority")
        n170 = event-data() -> ()  [unwired: 1 in, 6 out]
        n171 = call "Enqueue Element Array.vi"("priority"=w397, "queue index"=0, "error in"=w394, "master data"="程序参数保存", "queue in"=w395) -> ("error out"=w392:errorcluster, "queue out"=w393:T11)  [unwired: 5 in]
      }
      event "测试按钮": Value Change {
        w406 = u16 1 items=["HPRI"=1, "LPRI"=0] ("priority")
        n172 = event-data() -> ()  [unwired: 1 in, 6 out]
        n173 = property on="Main" class="TabCtl (严格)"("Value"=enum32{"主参数", "计算圆心参数 ", "测试效果"}."测试效果" ("Main")) -> ()  [unwired: 2 in, 2 out]
        n174 = call "Enqueue Element Array.vi"("priority"=w406, "queue index"=0, "error in"=w403, "master data"="测试按钮", "queue in"=w404) -> ("error out"=w401:errorcluster, "queue out"=w402:T11)  [unwired: 5 in]
        n175 = property on="计数器" class="DigNum (严格)"("Value"=200.0 ("计数器")) -> ()  [unwired: 2 in, 2 out]
      }
      event "启动200自动": Value Change {
        w415 = u16 1 items=["HPRI"=1, "LPRI"=0] ("priority")
        n176 = event-data() -> ()  [unwired: 1 in, 6 out]
        n177 = property on="Main" class="TabCtl (严格)"("Value"=enum32{"主参数", "计算圆心参数 ", "测试效果"}."测试效果" ("Main")) -> ()  [unwired: 2 in, 2 out]
        n178 = call "Enqueue Element Array.vi"("priority"=w415, "queue index"=0, "error in"=w412, "master data"="200自动", "queue in"=w413) -> ("error out"=w410:errorcluster, "queue out"=w411:T11)  [unwired: 5 in]
        n179 = local write "计数器"(0.0 ("计数器")) -> ()
      }
      event "采图按钮": Value Change {
        w425 = u16 1 items=["HPRI"=1, "LPRI"=0] ("priority")
        n180 = event-data() -> ()  [unwired: 1 in, 6 out]
        n181 = property on="Main" class="TabCtl (严格)"("Value"=enum32{"主参数", "计算圆心参数 ", "测试效果"}."测试效果" ("Main")) -> ()  [unwired: 2 in, 2 out]
        n182 = call "Enqueue Element Array.vi"("priority"=w425, "queue index"=0, "error in"=w422, "master data"="采图按钮", "queue in"=w423) -> ("error out"=w420:errorcluster, "queue out"=w421:T11)  [unwired: 5 in]
        n183 = property on="计数器" class="DigNum (严格)"("Value"=200.0 ("计数器")) -> ()  [unwired: 2 in, 2 out]
        n184 = local write "启动200自动"(FALSE ("启动200自动")) -> ()
      }
      event "获取ROI": Value Change {
        w433 = u16 1 items=["HPRI"=1, "LPRI"=0] ("priority")
        n185 = event-data() -> ()  [unwired: 1 in, 6 out]
        n186 = property on="Main" class="TabCtl (严格)"("Value"=enum32{"主参数", "计算圆心参数 ", "测试效果"}."测试效果" ("Main")) -> ()  [unwired: 2 in, 2 out]
        n187 = call "Enqueue Element Array.vi"("priority"=w433, "queue index"=0, "error in"=w430, "master data"="获取ROI", "queue in"=w431) -> ("error out"=w428:errorcluster, "queue out"=w429:T11)  [unwired: 5 in]
      }
      event "200测试": Value Change {
        w441 = u16 1 items=["HPRI"=1, "LPRI"=0] ("priority")
        n188 = event-data() -> ()  [unwired: 1 in, 6 out]
        n189 = property on="Main" class="TabCtl (严格)"("Value"=enum32{"主参数", "计算圆心参数 ", "测试效果"}."测试效果" ("Main")) -> ()  [unwired: 2 in, 2 out]
        n190 = call "Enqueue Element Array.vi"("priority"=w441, "queue index"=0, "error in"=w438, "master data"="200测试", "queue in"=w439) -> ("error out"=w436:errorcluster, "queue out"=w437:T11)  [unwired: 5 in]
      }
      event "GRR测试": Value Change {
        w449 = u16 1 items=["HPRI"=1, "LPRI"=0] ("priority")
        n191 = event-data() -> ()  [unwired: 1 in, 6 out]
        n192 = property on="Main" class="TabCtl (严格)"("Value"=enum32{"主参数", "计算圆心参数 ", "测试效果"}."测试效果" ("Main")) -> ()  [unwired: 2 in, 2 out]
        n193 = call "Enqueue Element Array.vi"("priority"=w449, "queue index"=0, "error in"=w446, "master data"="GRR测试", "queue in"=w447) -> ("error out"=w444:errorcluster, "queue out"=w445:T11)  [unwired: 5 in]
      }
      event "刷新": Value Change {
        n194 = event-data() -> ()  [unwired: 1 in, 6 out]
        n195 = disable-structure shown="禁用" {
          disable-tunnel: w455 -> [w459 _]
          disable-tunnel: w454 -> [w458 _]
          disable-tunnel: [w457 _] -> w453
          disable-tunnel: [w456 _] -> w452
          frame Disabled {
            w461 = u16 1 items=["HPRI"=1, "LPRI"=0] ("priority")
            # "刷新"
            n196 = call "Enqueue Element Array.vi"("priority"=w461, "queue index"=0, "error in"=w458, "master data"="刷新", "queue in"=w459) -> ("error out"=w456:errorcluster, "queue out"=w457:T11)  [unwired: 5 in]
          }
          frame Enabled {
          }
        }
        n197 = property on="Main" class="TabCtl (严格)"("Value"=enum32{"主参数", "计算圆心参数 ", "测试效果"}."主参数" ("Main")) -> ()  [unwired: 2 in, 2 out]
      }
    }
    n198 = call "GetSystemTime.vi"() -> ("date/time string"=→"system time":string)  [unwired: 7 in]
  }
  n199 = call "Release Queue Array.vi"("error in"=w5, "queue in"=w3) -> ("error out"=w4:errorcluster)  [unwired: 2 in, 3 out]
  n200 = call "Release Queue Array.vi"("error in"=w8, "queue in"=w3) -> ("error out"=w11:errorcluster)  [unwired: 2 in, 3 out]
  n201 = call "MergeErrors.vi"("error in 3 (no error)"=w4, "error in 4 (no error)"=w11) -> ("error out"=w10:errorcluster)  [unwired: 6 in]
  n202 = disable-structure shown="启用" {
    disable-tunnel: w10 -> [w464 w465]
    disable-tunnel: [w463 w465] -> w9
    frame Disabled {
      n203 = call "ExitAppMode.vi"("error in (no error)"=w464) -> ("error out"=w463:errorcluster)  [unwired: 10 in]
    }
    frame Enabled {
    }
  }
  n204 = call <vilib>:"Clear Errors.vi"("error in (no error)"=w9) -> ()  [unwired: 5 in, 2 out]
  "计数器" <- 0.0 ("数值")
